vi "Read Pressure Servo Valve Settings.vi"(8 "error in (no error)":errorcluster, 11 "Boot Loader in":refnum<class "Boot Loader.lvclass">) -> (0 "error out":errorcluster, 2 "Pressure Servo Valve Settings":T1={"Center Point"=2.5, "Area"=0.004536, "PA to PSI"=0.000145038, "Off Value"=0.004536} {"Off Value" format="%.3f"; "PA to PSI" format="%.9f"; "Area" format="%.9f"; "Center Point" format="%.3f"}, 3 "Boot Loader out":refnum<class "Boot Loader.lvclass">)   [LabVIEW 2015, in "Boot Loader.lvclass"]
uses:
  Boot Loader.lvclass
  Typedefs/Pressure Servo Valve Settings.ctl
  Settings/Settings.lvclass
  Typedefs/FAMT Typedefs.lvlib
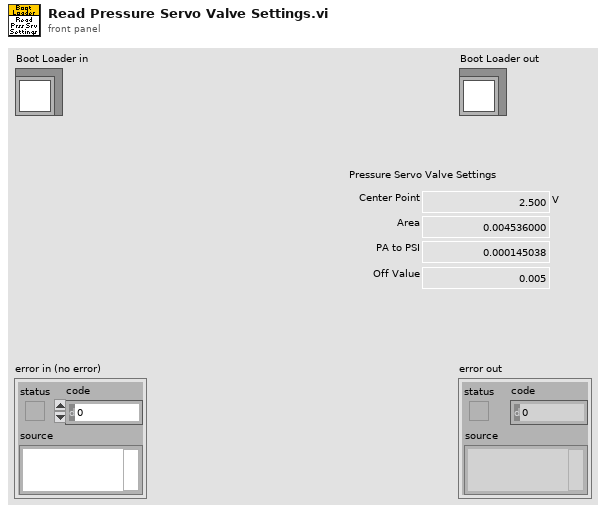
[diagram p1: front panel]
types:
  T1 = typedef "FAMT Typedefs.lvlib/Pressure Servo Valve Settings.ctl" = cluster{"Center Point":dbl[unit], "Area":dbl, "PA to PSI":dbl, "Off Value":dbl}
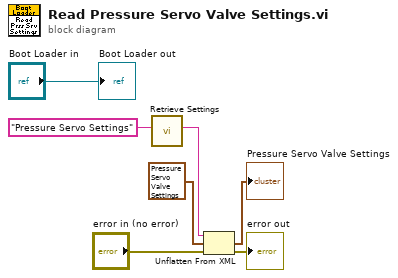
[diagram p0: block diagram]
diagram:
  n1 = call "Retrieve Settings.vi"("configName"="Pressure Servo Settings") -> ("xmlConfig"=w5:string)  [unwired: 8 in, 2 out]
  n2 = Unflatten From XML(xml string=w5, type=T1 {"Center Point"=2.5, "Area"=0.004536, "PA to PSI"=0.000145038, "Off Value"=0.004536} ("Pressure Servo Valve Settings"), error in (no error)="error in (no error)") -> (value=→"Pressure Servo Valve Settings":T1, error out=→"error out":errorcluster)
  "Boot Loader out" <- "Boot Loader in"
